vi "Reconnect.vi"(8 "error in (With error)":errorcluster={"status"=TRUE, "code"=0, "source"=""}, 11 "Hardware in":refnum<class "Hardware.lvclass">) -> (0 "error out":errorcluster, 2 "Reconnected":bool, 3 "Hardware out":refnum<class "Hardware.lvclass">)   [LabVIEW 2016, in "Hardware.lvlib" / "Hardware.lvclass"]
uses:
  <userlib>/Common Components/Hardware/Abstract Hardware/Hardware.lvclass
panel:
  # "This VI is only called on error!"
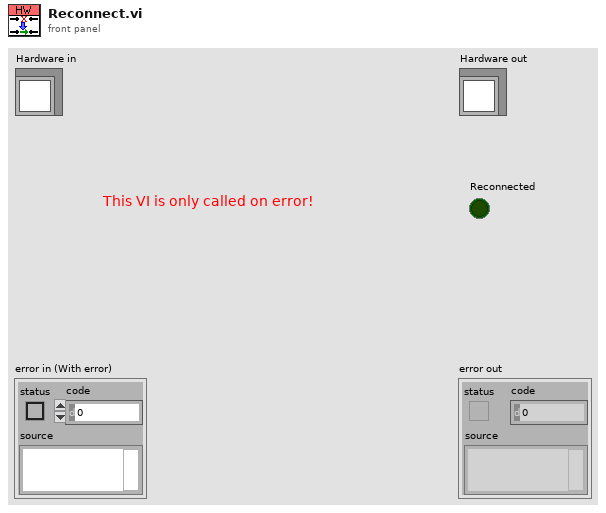
[diagram p1: front panel]
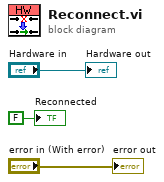
[diagram p0: block diagram]
diagram:
  "error out" <- "error in (With error)"
  "Hardware out" <- "Hardware in"
  "Reconnected" <- FALSE ("Reconnected")
